vi "JJMCclase7trabajo2.vi"() -> ()   [LabVIEW 2011]
panel:
  out "contador":dbl
  out "menor":dbl
  out "mayor":dbl
  out "promedio":dbl
  out "Thermometer":i32(slide) scale=0.0..100.0
  # "genrar 10 temperaturas y al finalpresentar la temperatura mayor, menor y la temperatura promedio"
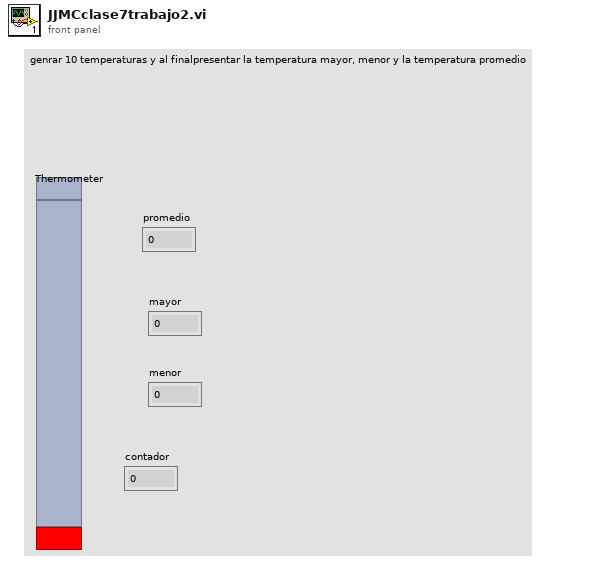
[diagram p1: front panel]
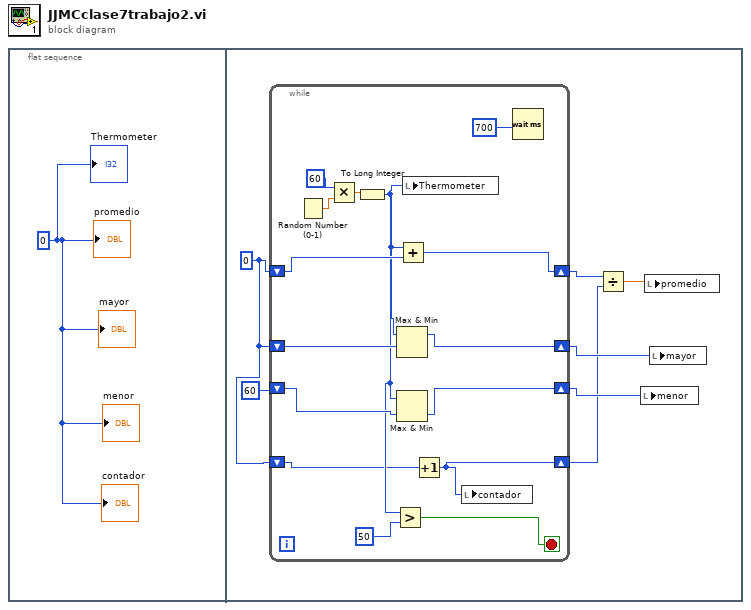
[diagram p0: block diagram]
diagram:
  n1 = flat-sequence {
    frame #0 {
      w1 = 0
      "Thermometer" <- w1
      "promedio" <- w1
      "mayor" <- w1
      "menor" <- w1
      "contador" <- w1
    }
    frame #1 {
      w3 = 0
      n2 = while {
        shift-right: [w20] -> w8
        shift-left: w3 -> [w19]
        shift-right: [w16] -> w6
        shift-left: w3 -> [w17]
        shift-right: [w14] -> w5
        shift-left: 60 -> [w15]
        shift-right: [w9] -> w2
        shift-left: w3 -> [w10]
        stop <- w11 stop-if-true
        n3 = Random Number (0-1)() -> (number: 0 to 1=w23:dbl)
        n4 = Multiply(x=60, y=w23) -> (x*y=w22:dbl)
        n5 = To Long Integer(number=w22) -> (32bit integer=w12:i32)
        n6 = Greater?(x=w12, y=50) -> (0:w11:bool)
        n7 = Max & Min(x=w12, y=w17) -> (max(x,y)=w16:i32)  [unwired: 1 out]
        n8 = Max & Min(x=w12, y=w15) -> (min(x,y)=w14:i32)  [unwired: 1 out]
        n9 = Add(x=w12, y=w19) -> (x+y=w20:i32)
        n10 = local write "Thermometer"(w12) -> ()
        n11 = Increment(x=w10) -> (x+1=w9:i32)
        n12 = local write "contador"(w9) -> ()
        n13 = Wait (ms)(milliseconds to wait=700) -> ()  [unwired: 1 out]
      }
      n14 = Divide(x=w8, y=w2) -> (x/y=w7:dbl)
      n15 = local write "menor"(w5) -> ()
      n16 = local write "promedio"(w7) -> ()
      n17 = local write "mayor"(w6) -> ()
    }
  }
